vi "_RT_CtrlLoop_SigTrnsfr_Process.vi"(8 "error in (no error)":errorcluster, 10 "system state":refnum<data-value>, 11 "Signal Queue Input":refnum<queue>) -> (0 "error out":errorcluster)   [LabVIEW 2018]
uses:
  PublicSubVI/Ctl/_ctl_RT_System_State.ctl
  PublicSubVI/Ctl/_ctl_RT_SysLog.ctl
  <resource>/objmgr/ni.dex.rc
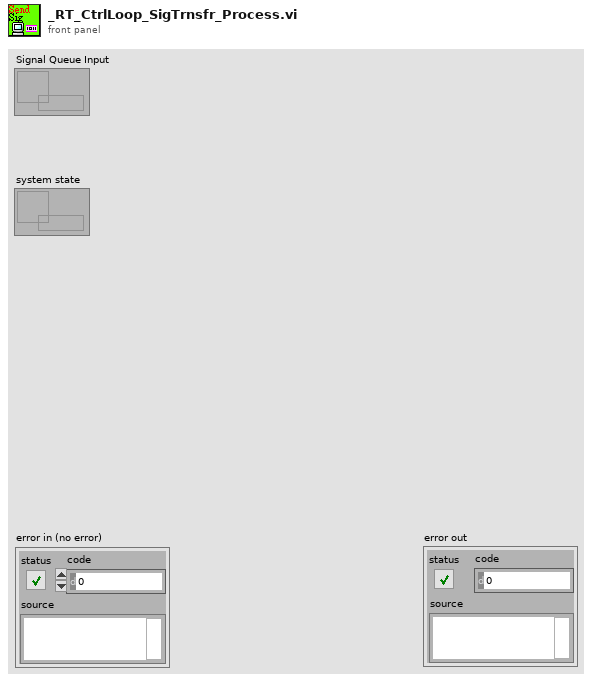
[diagram p1: front panel]
types:
  T1 = typedef "_ctl_RT_SysLog.ctl" = enum16{"None", "Initialize", "StartupRT", "StartupFPGA", "StartupAllocator", "GetMass", "SetWfmCode", "SetLaserCtrl", "SetTurboCtrl", "SetD999Ctrl", "Reconnecting...", "Interrupt", "StopRT"}
  T2 = typedef "_ctl_RT_System_State.ctl" = enum16{"initialize", "idle", "working", "disconnect"}
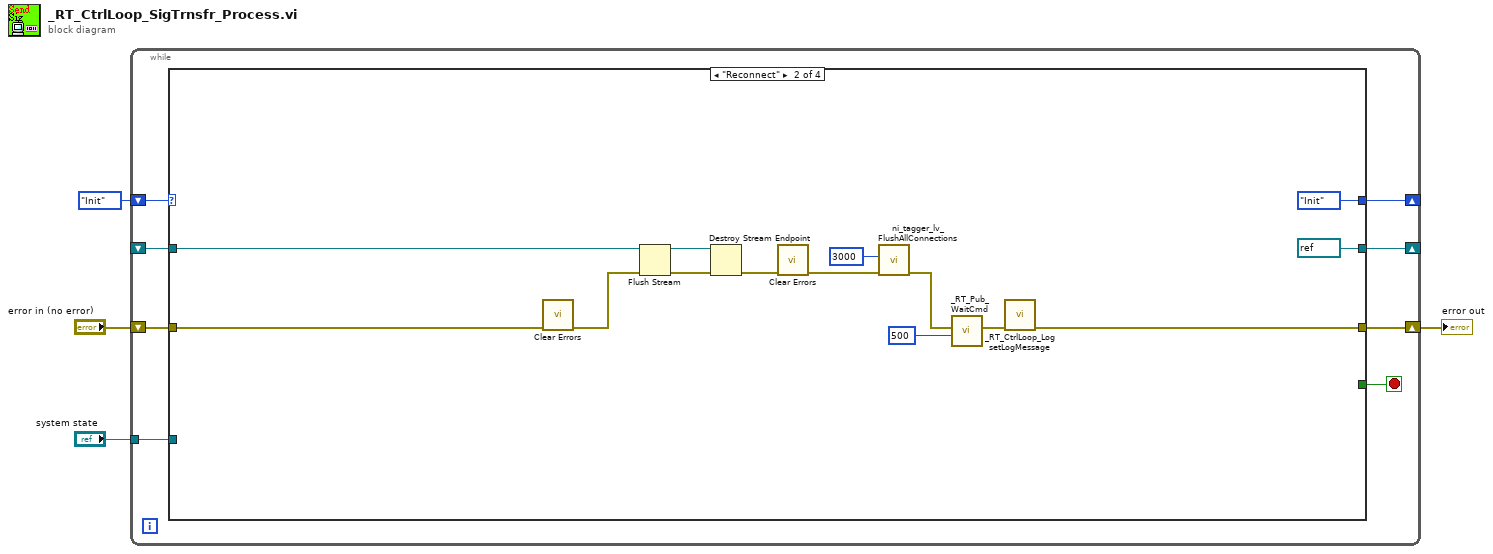
[diagram p0: block diagram]
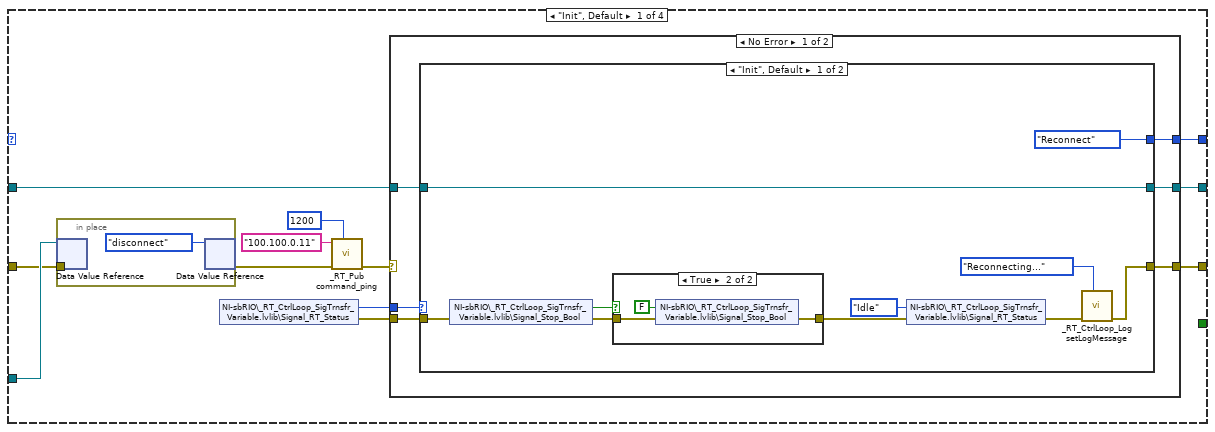
[diagram p2: hidden frame]
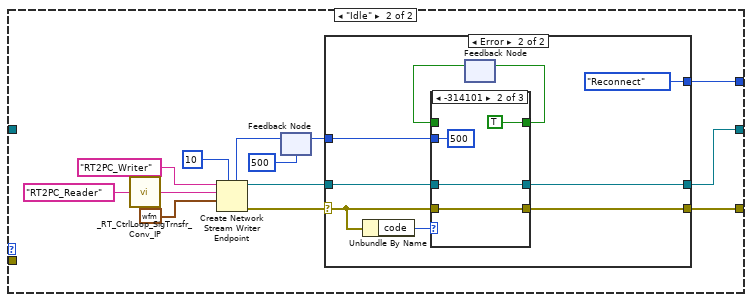
[diagram p4: hidden frame]
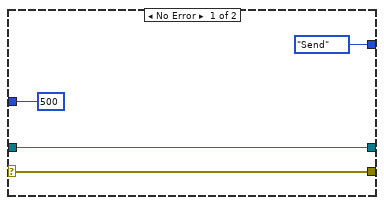
[diagram p5: hidden frame]
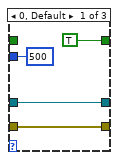
[diagram p6: hidden frame]
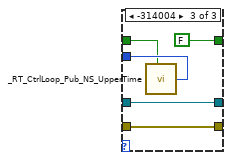
[diagram p7: hidden frame]
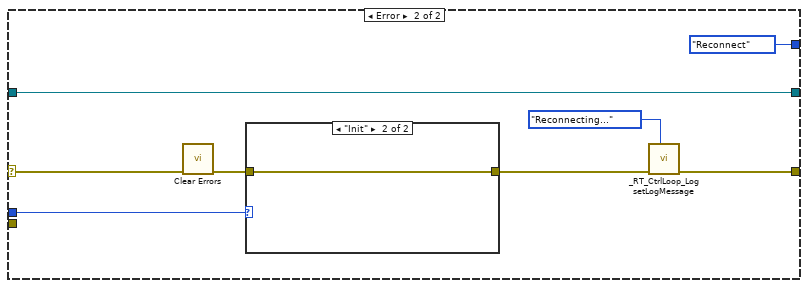
[diagram p8: hidden frame]
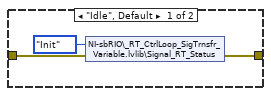
[diagram p9: hidden frame]
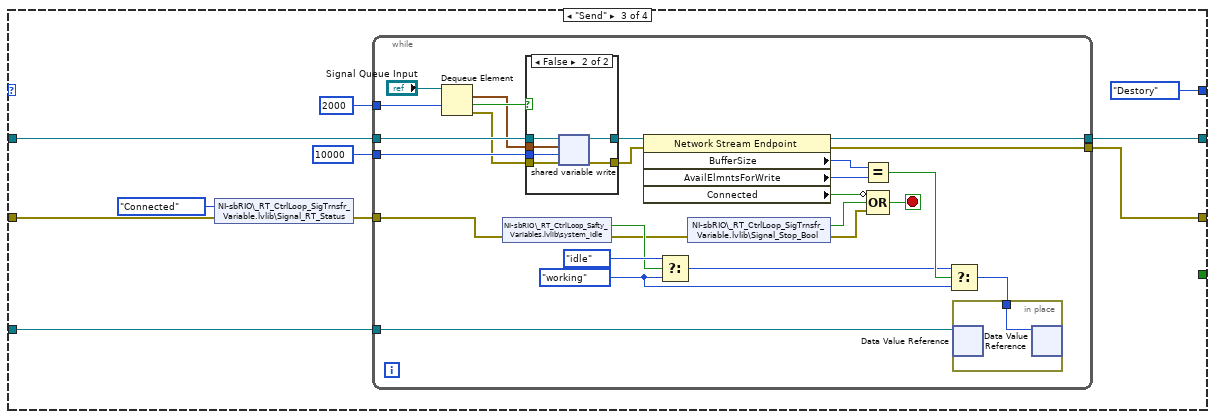
[diagram p10: hidden frame]
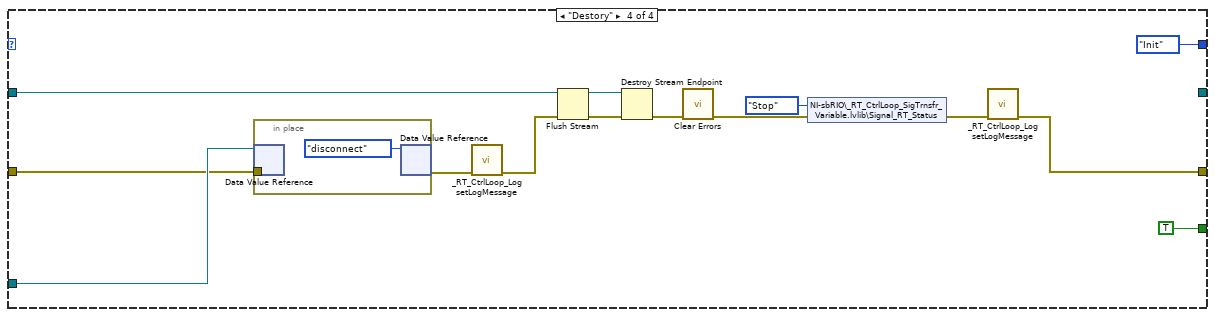
[diagram p12: hidden frame]
diagram:
  n1 = while {
    shift-right: [w12] -> _
    shift-left: _ -> [w11]
    shift-right: [w10] -> _
    shift-left: enum8{"Init", "Reconnect", "Send", "Destory"}."Init" -> [w5]
    tunnel: "system state" -> [w8]
    shift-right: [w6] -> w3
    shift-left: "error in (no error)" -> [w7]
    stop <- w9 stop-if-true
    n2 = case shown="\"Reconnect\"" w5 {
      tunnel: [w24 refnum<k21> refnum ("writer name") w119 _] -> w12
      tunnel: w7 -> [w21 w100 w116 w164]
      tunnel: [w23 w102 w118 w159] -> w6
      tunnel: w11 -> [w13 w104 w120 w163]
      tunnel: [w14 enum8{"Init", "Reconnect", "Send", "Destory"}."Init" enum8{"Init", "Reconnect", "Send", "Destory"}."Destory" ("f") enum8{"Init", "Reconnect", "Send", "Destory"}."Init" ("f")] -> w10
      tunnel: [_ _ _ TRUE ("Boolean")] -> w9
      tunnel: w8 -> [w22 _ w117 w168]
      frame "Init", Default {
        n3 = in-place {
          in-place-border: w21 -> [_]
          n4 = in-place-dvr #1(w22) -> ()  [unwired: 2 out]
          n5 = in-place-dvr #1(_ctl_RT_System_State."disconnect" ("data value")) -> (w18:errorcluster)  [unwired: 1 out]
        }
        n6 = shared-variable "NI-sbRIO\\_RT_CtrlLoop_SigTrnsfr_Variable.lvlib\\Signal_RT_Status"() -> (w16:enum8{"Idle", "Init", "Connected", "Stop"}, error out=w15:errorcluster)  [unwired: 1 in]
        n7 = call "_RT_Pub command_ping.vi"("Loop Times"=1200, "error in (no error)"=w18, "PCIP String"="100.100.0.11") -> ("error out"=w17:errorcluster)  [unwired: 8 in]
        n8 = case shown="No Error" w17 {
          selector: w17 -> [_ w91]
          tunnel: [w30 w84] -> w24
          tunnel: [w29 w85] -> w23
          tunnel: w16 -> [w27 w89]
          tunnel: w15 -> [w28 _]
          tunnel: [w26 enum8{"Init", "Reconnect", "Send", "Destory"}."Reconnect"] -> w14
          tunnel: w13 -> [w25 w84]
          frame No Error {
            n9 = case shown="\"Init\", Default" w27 {
              tunnel: [w31 w47] -> w30
              tunnel: [w33 w46] -> w29
              tunnel: w28 -> [w38 _]
              tunnel: [enum8{"Init", "Reconnect", "Send", "Destory"}."Reconnect" ("f") w45] -> w26
              tunnel: w25 -> [w31 _]
              frame "Init", Default {
                n10 = shared-variable "NI-sbRIO\\_RT_CtrlLoop_SigTrnsfr_Variable.lvlib\\Signal_Stop_Bool"(error in=w38) -> (w40:bool, error out=w39:errorcluster)
                n11 = case shown="True" w40 {
                  tunnel: w39 -> [w41 w43]
                  tunnel: [w41 w42] -> w37
                  frame False {
                  }
                  frame True {
                    n12 = shared-variable "NI-sbRIO\\_RT_CtrlLoop_SigTrnsfr_Variable.lvlib\\Signal_Stop_Bool"(FALSE ("Signal_Stop_Bool"), error in=w43) -> (error out=w42:errorcluster)
                  }
                }
                n13 = shared-variable "NI-sbRIO\\_RT_CtrlLoop_SigTrnsfr_Variable.lvlib\\Signal_RT_Status"(enum8{"Idle", "Init", "Connected", "Stop"}."Idle" ("Signal_RT_Status"), error in=w37) -> (error out=w35:errorcluster)
                n14 = call "_RT_CtrlLoop_Log setLogMessage.vi"("system type"=_ctl_RT_SysLog."Reconnecting...", "error in"=w35) -> ("error out"=w33:errorcluster)  [unwired: 8 in, 1 out]
              }
              frame "Idle" {
                n15 = call "_RT_CtrlLoop_SigTrnsfr_Conv_IP.vi"("EndPoint"="RT2PC_Reader" ("reader url")) -> ("IP/Endpoint"=w54:string)
                n16 = feedback #2(500 ("UpdateTime")) -> (w57:i32)
                n17 = Create Network Stream Writer Endpoint(5:w57, 7:10 ("writer buffer size"), 9:waveform(i16) {"t0"=timestamp(0 s since 1904-01-01), "dt"=1.0, "Y"=[]} ("element"), 10:w54, 11:"RT2PC_Writer" ("writer name")) -> (0:w56:errorcluster, 3:w55:refnum<k21>)  [unwired: 2 in]
                n18 = case shown="Error" w56 {
                  selector: w56 -> [w60 w68]
                  tunnel: [w61 w69] -> w47
                  tunnel: [w60 w63] -> w46
                  tunnel: w55 -> [w61 w66]
                  tunnel: [500 ("UpdateTime") w67] -> w48
                  tunnel: [enum8{"Init", "Reconnect", "Send", "Destory"}."Send" ("f") enum8{"Init", "Reconnect", "Send", "Destory"}."Reconnect"] -> w45
                  frame No Error {
                  }
                  frame Error {
                    n19 = Unbundle By Name(w68) -> ("code"=w70:i32)
                    n20 = feedback #3() -> (w64:bool)  [unwired: 1 in]
                    n21 = case shown="-314101" w70 {
                      tunnel: [w72 w78 w82] -> w69
                      tunnel: w66 -> [w72 w78 w82]
                      tunnel: [w74 w77 w79] -> w63
                      tunnel: w68 -> [w74 w77 w79]
                      tunnel: w64 -> [_ _ w81]
                      tunnel: [500 ("UpdateTime") 500 ("UpdateTime") w83] -> w67
                      tunnel: [TRUE TRUE FALSE] -> w65
                      frame 0, Default {
                      }
                      frame -314101 {
                      }
                      frame -314004 {
                        n22 = call "_RT_CtrlLoop_Pub_NS_UpperTime.vi"("Init? (F)"=w81) -> ("UpdateTime"=w83:i32)  [unwired: 4 in]
                      }
                    }
                    n23 = feedback-in #3(w65) -> ()
                  }
                }
                n24 = feedback-in #2(w48) -> ()
              }
            }
          }
          frame Error {
            n25 = call <vilib>:"Clear Errors.vi"("error in (no error)"=w91) -> ("error out"=w90:errorcluster)  [unwired: 5 in, 1 out]
            n26 = case shown="\"Init\"" w89 {
              tunnel: w90 -> [w93 w95]
              tunnel: [w92 w95] -> w87
              frame "Idle", Default {
                n27 = shared-variable "NI-sbRIO\\_RT_CtrlLoop_SigTrnsfr_Variable.lvlib\\Signal_RT_Status"(enum8{"Idle", "Init", "Connected", "Stop"}."Init" ("Signal_RT_Status"), error in=w93) -> (error out=w92:errorcluster)
              }
              frame "Init" {
              }
            }
            n28 = call "_RT_CtrlLoop_Log setLogMessage.vi"("system type"=_ctl_RT_SysLog."Reconnecting...", "error in"=w87) -> ("error out"=w85:errorcluster)  [unwired: 8 in, 1 out]
          }
        }
      }
      frame "Reconnect" {
        n29 = call <vilib>:"Clear Errors.vi"("error in (no error)"=w100) -> ("error out"=w99:errorcluster)  [unwired: 5 in, 1 out]
        n30 = Flush Stream(8:w99, 11:w104) -> (0:w108:errorcluster, 3:w107:refnum<k21>)  [unwired: 2 in, 1 out]
        n31 = Destroy Stream Endpoint(8:w108, 11:w107) -> (0:w98:errorcluster)
        n32 = call <vilib>:"Clear Errors.vi"("error in (no error)"=w98) -> ("error out"=w97:errorcluster)  [unwired: 5 in, 1 out]
        n33 = call <vilib>:"ni_tagger_lv_FlushAllConnections.vi"("error in (no error)"=w97, "timeout ms (1000)"=3000) -> ("error out"=w106:errorcluster)  [unwired: 8 in, 1 out]
        n34 = call "_RT_Pub_WaitCmd.vi"("milliseconds to wait"=u32 500, "error in (no error)"=w106) -> ("error out"=w103:errorcluster)  [unwired: 9 in]
        n35 = call "_RT_CtrlLoop_Log setLogMessage.vi"("error in"=w103) -> ("error out"=w102:errorcluster)  [unwired: 9 in, 1 out]
      }
      frame "Send" {
        n36 = shared-variable "NI-sbRIO\\_RT_CtrlLoop_SigTrnsfr_Variable.lvlib\\Signal_RT_Status"(enum8{"Idle", "Init", "Connected", "Stop"}."Connected" ("Signal_RT_Status"), error in=w116) -> (error out=w114:errorcluster)
        n37 = while {
          tunnel: w120 -> [w146]
          tunnel: w114 -> [w123]
          tunnel: w117 -> [w121]
          tunnel: 2000 ("timeout in ms (-1)") -> [w139]
          tunnel: 10000 ("timeout in ms (-1)") -> [w138]
          tunnel: [w134] -> w119
          tunnel: [w133] -> w118
          stop <- w141 stop-if-true
          w124 = _ctl_RT_System_State."working" ("data value")
          n38 = Dequeue Element(queue="Signal Queue Input", timeout in ms (-1)=w139) -> (element=w143:waveform(i16), timed out?=w145:bool, error out=w137:errorcluster)  [unwired: 1 in, 1 out]
          n39 = shared-variable "NI-sbRIO\\_RT_CtrlLoop_Safty_Variables.lvlib\\system_idle"(error in=w123) -> (w127:bool, error out=w126:errorcluster)
          n40 = case shown="False" w145 {
            tunnel: w146 -> [w149 w155]
            tunnel: w137 -> [w148 w154]
            tunnel: [w149 w153] -> w136
            tunnel: [w148 w152] -> w135
            tunnel: w143 -> [_ w151]
            tunnel: w138 -> [_ w150]
            frame True {
            }
            frame False {
              n41 = shared-variable-write(w155, w154, w151, w150) -> (w153:refnum<k21>, w152:errorcluster)  [unwired: 1 out]
            }
          }
          n42 = property class="Network Stream Endpoint"(reference=w136, error in=w135) -> (reference out=w134:refnum<k21>, error out=w133:errorcluster, "BufferSize"=w132:i32, "AvailElmntsForWrite"=w131:i32, "Connected"=w130:bool)
          n43 = Select(t=_ctl_RT_System_State."idle" ("data value"), s=w127, f=w124) -> (s? t:f=w125:T2)
          n44 = shared-variable "NI-sbRIO\\_RT_CtrlLoop_SigTrnsfr_Variable.lvlib\\Signal_Stop_Bool"(error in=w126) -> (w142:bool, error out=w140:errorcluster)
          n45 = Equal?(x=w132, y=w131) -> (x = y?=w129:bool)
          n46 = Compound Arithmetic op=OR(invert w130, w142, w140) -> (w141:bool)
          n47 = Select(t=w125, s=w129, f=w124) -> (s? t:f=w122:T2)
          n48 = in-place {
            in-place-border: w122 -> [w147]
            n49 = in-place-dvr #4(w121) -> ()  [unwired: 2 out]
            n50 = in-place-dvr #4(w147) -> ()  [unwired: 2 out]
          }
        }
      }
      frame "Destory" {
        n51 = in-place {
          in-place-border: w164 -> [_]
          n52 = in-place-dvr #5(w168) -> ()  [unwired: 2 out]
          n53 = in-place-dvr #5(_ctl_RT_System_State."disconnect" ("data value")) -> (w157:errorcluster)  [unwired: 1 out]
        }
        n54 = call "_RT_CtrlLoop_Log setLogMessage.vi"("error in"=w157) -> ("error out"=w156:errorcluster)  [unwired: 9 in, 1 out]
        n55 = Flush Stream(8:w156, 11:w163) -> (0:w161:errorcluster, 3:w162:refnum<k21>)  [unwired: 2 in, 1 out]
        n56 = Destroy Stream Endpoint(8:w161, 11:w162) -> (0:w169:errorcluster)
        n57 = call <vilib>:"Clear Errors.vi"("error in (no error)"=w169) -> ("error out"=w165:errorcluster)  [unwired: 5 in, 1 out]
        n58 = shared-variable "NI-sbRIO\\_RT_CtrlLoop_SigTrnsfr_Variable.lvlib\\Signal_RT_Status"(enum8{"Idle", "Init", "Connected", "Stop"}."Stop" ("Signal_RT_Status"), error in=w165) -> (error out=w160:errorcluster)
        n59 = call "_RT_CtrlLoop_Log setLogMessage.vi"("error in"=w160) -> ("error out"=w159:errorcluster)  [unwired: 9 in, 1 out]
      }
    }
  }
  "error out" <- w3
